vi "RenameWorksheet.vi"(8 "error in (no error)":errorcluster, 9 "New Worksheet Name":string="Worksheet New Name", 10 "Worksheet Index":i32, 11 "ExcelFile in":refnum<class "PortableExcelFileManipulationOXML.lvclass">) -> (0 "error out":errorcluster, 3 "ExcelFile out":refnum<class "PortableExcelFileManipulationOXML.lvclass">)   [LabVIEW 2019, in "PortableExcelFileManipulationOXML.lvclass"]
uses:
  PortableExcelFileManipulationOXML.lvclass
  PortableExcelFileManipulationOXML.lvclass/PortableExcelFileManipulationOXML.ctl
  H:/LV projects/ExpressionEvaluator/Excel/ExcelManipulation.dll
  ExcelManipulation.dll
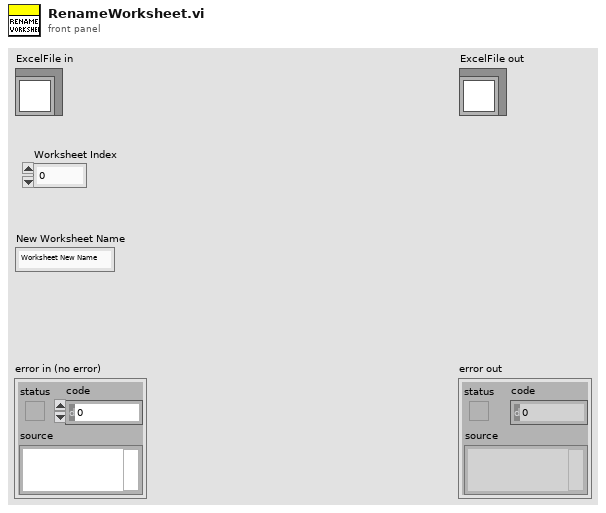
[diagram p1: front panel]
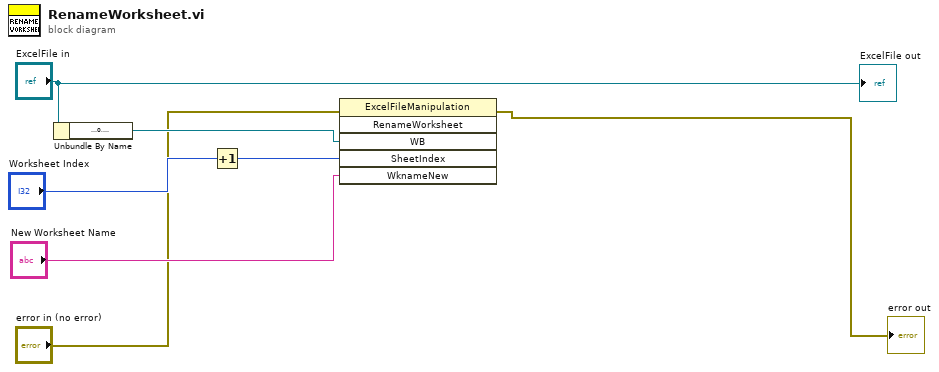
[diagram p0: block diagram]
diagram:
  n1 = Unbundle By Name("ExcelFile in") -> ("ExcelOpen"=w6:refnum<k24>)
  n2 = Increment(x="Worksheet Index") -> (x+1=w1:i32)
  n3 = invoke class="ExcelFileManipulation" method="RenameWorksheet"(error in="error in (no error)", "WB"=w6, "SheetIndex"=w1, "WknameNew"="New Worksheet Name") -> (error out=→"error out":errorcluster)  [unwired: 2 in, 5 out]
  "ExcelFile out" <- "ExcelFile in"
